vi "SeCrTS-DI Index FGV .vi"(7 "Action":enum16{"Write", "Read", "Init"}(ring), 11 "Ai Index Element":i32[](array[numeric])) -> (3 "Ai Index Element R":i32[](array[numeric]))   [LabVIEW 2022 SP3]
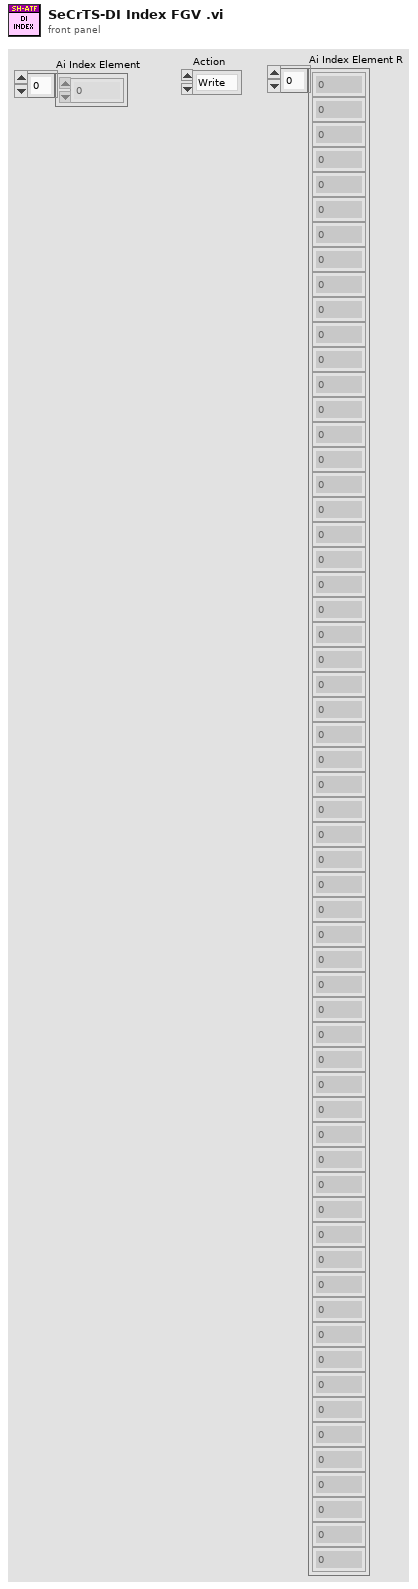
[diagram p1: front panel]
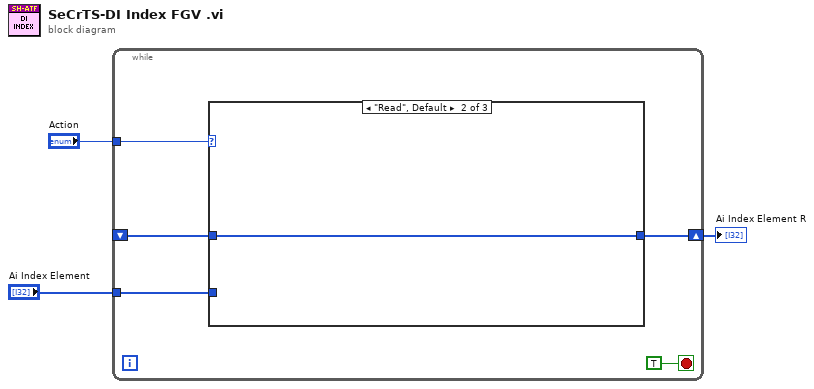
[diagram p0: block diagram]
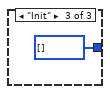
[diagram p3: hidden frame]
diagram:
  n1 = while {
    tunnel: "Action" -> [w8]
    shift-right: [w6] -> w1
    shift-left: _ -> [w7]
    tunnel: "Ai Index Element" -> [w5]
    stop <- TRUE stop-if-true
    n2 = case shown="\"Read\", Default" w8 {
      tunnel: w7 -> [_ w10 _]
      tunnel: [w9 w10 i32[] [] ("Ai Index Element")] -> w6
      tunnel: w5 -> [w9 _ _]
      frame "Write" {
      }
      frame "Read", Default {
      }
      frame "Init" {
      }
    }
  }
  "Ai Index Element R" <- w1
